vi "Script Example Project.vi"(8 "Error In":errorcluster, 10 "Hostname or IP":string="192.168.7.2", 11 "Device Name":string="BeagleBone Black") -> (0 "Error Out":errorcluster)   [LabVIEW 2019, in "LMH-LINX.lvlib"]
uses:
  <vilib>/MakerHub/LINX/LMH-LINX.lvlib
  <vilib>/MakerHub/Toolbox/LMH-Toolbox.lvlib
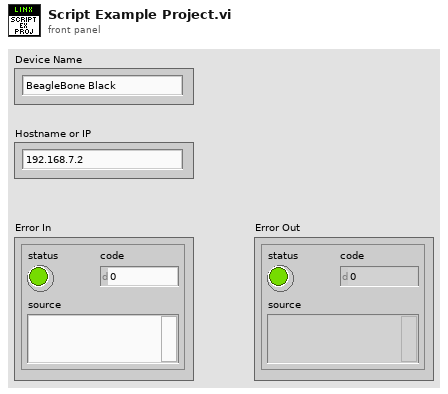
[diagram p1: front panel]
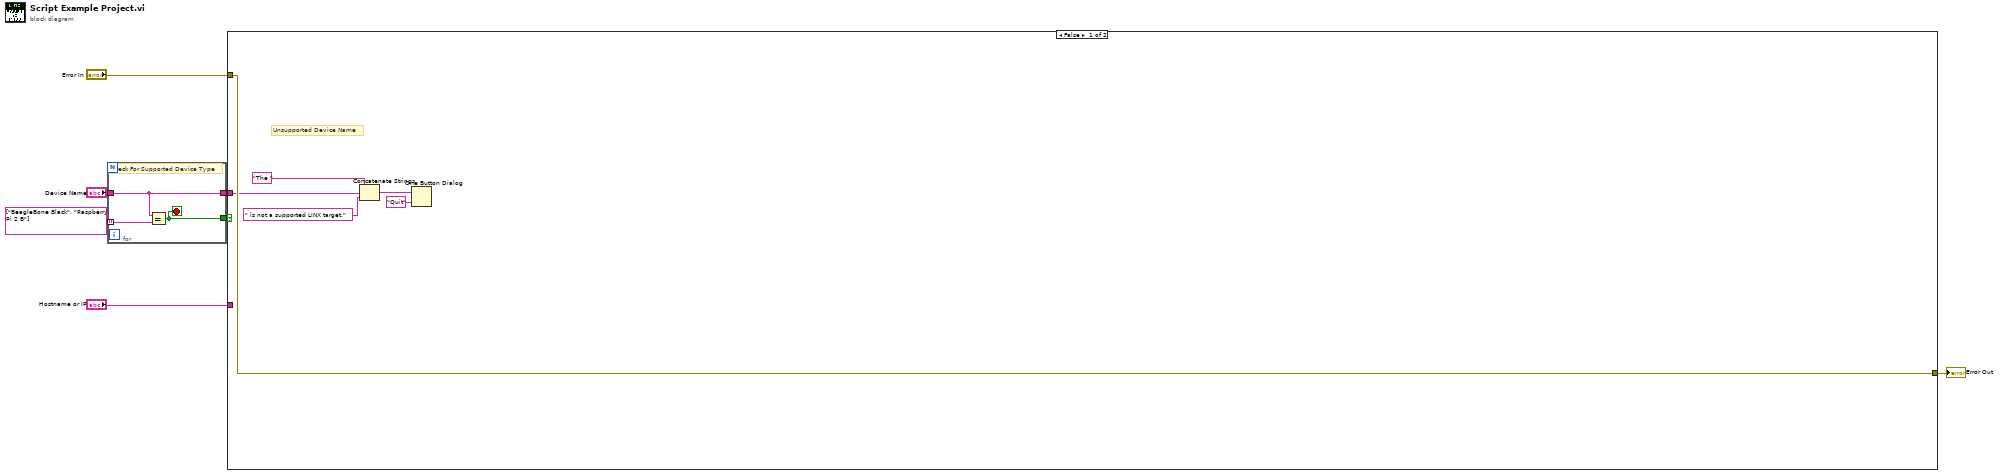
[diagram p0: block diagram]
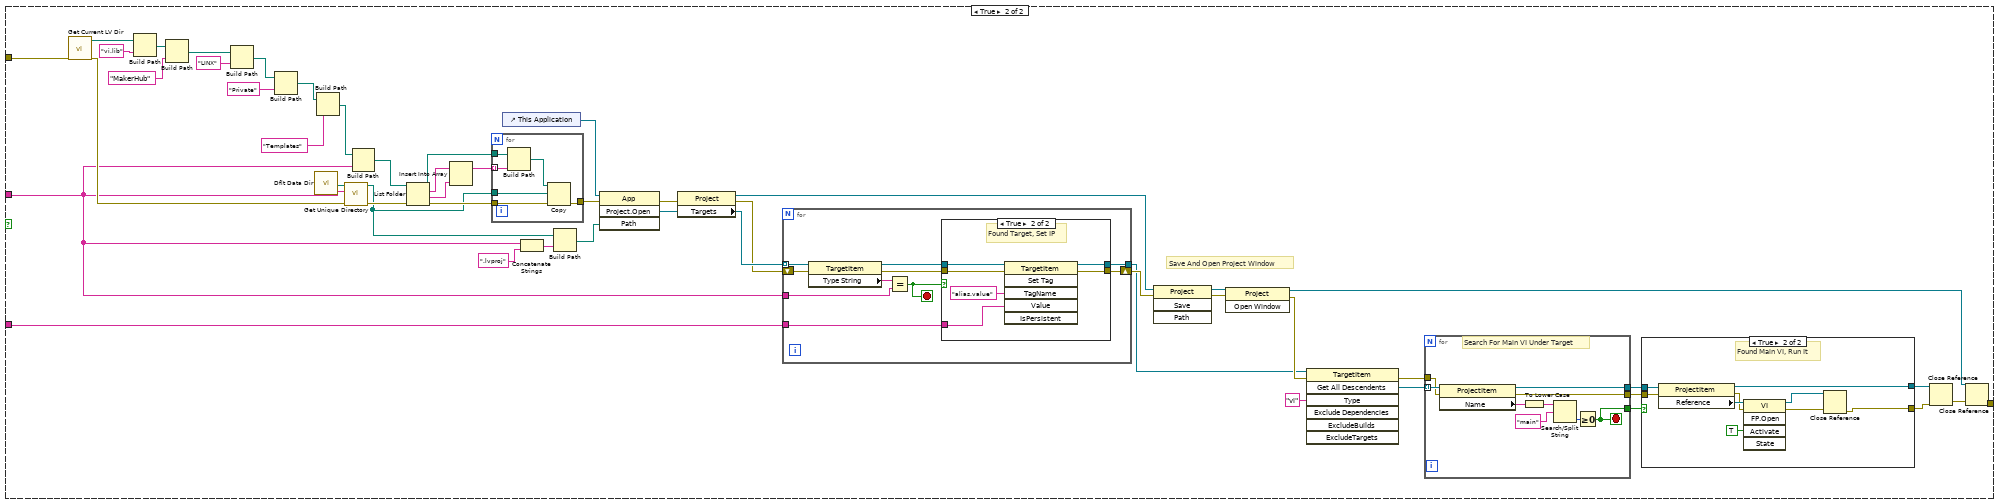
[diagram p2: hidden frame]
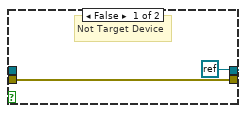
[diagram p4: hidden frame]
diagram:
  n1 = for {
    tunnel: string[] ["BeagleBone Black", "Raspberry Pi 2 B"] -> [w10] mode=indexing
    tunnel: "Device Name" -> [w8]
    tunnel: [w9] -> w1
    tunnel: [w8] -> w2
    stop <- w9 stop-if-true
    # "Check For Supported Device Type"
    n2 = Equal?(x=w8, y=w10) -> (x = y?=w9:bool)
  }
  n3 = case shown="False" w1 {
    tunnel: "Hostname or IP" -> [_ w53]
    tunnel: "Error In" -> [w16 w19]
    tunnel: [w16 w18] -> w5
    tunnel: w2 -> [w14 w17]
    frame False {
      # "Unsupported Device Name"
      n4 = Concatenate Strings("The " ("message"), w14, " is not a supported LINX target." ("string")) -> (w12:string)
      n5 = One Button Dialog(message=w12, button name ("OK")="Quit") -> ()  [unwired: 1 out]
    }
    frame True {
      # "Save And Open Project Window"
      n6 = call <vilib>:"Get Current LV Dir.vi"("Error In"=w19) -> ("Error Out"=w21:errorcluster, "This LV Directory"=w66:path)  [unwired: 9 in]
      n7 = Build Path(base path=w66, name or relative path="vi.lib") -> (appended path=w60:path)
      n8 = Build Path(base path=w60, name or relative path="MakerHub") -> (appended path=w59:path)
      n9 = Build Path(base path=w59, name or relative path="LINX") -> (appended path=w58:path)
      n10 = Build Path(base path=w58, name or relative path="Private") -> (appended path=w57:path)
      n11 = call <vilib>:"Dflt Data Dir.vi"() -> ("App:Default Data Directory"=w43:path)
      n12 = Build Path(base path=w57, name or relative path="Templates") -> (appended path=w56:path)
      n13 = call <vilib>:"Get Unique Directory.vi"("Error In"=w21, "Root Folder Name"=w17, "Parent Directory"=w43) -> ("Error Out"=w40:errorcluster, "Target Directory"=w35:path)  [unwired: 7 in]
      n14 = Build Path(base path=w56, name or relative path=w17) -> (appended path=w42:path)
      n15 = List Folder(path=w42, error in=w40) -> (path out=w37:path, filenames=w20:string[], folder names=w39:string[], error out=w41:errorcluster)  [unwired: 2 in]
      n16 = Insert Into Array(array=w20, new element=w39) -> (w38:string[])  [unwired: 1 in]
      n17 = for {
        tunnel: w41 -> [w92]
        tunnel: w38 -> [w91] mode=indexing
        tunnel: w37 -> [w90]
        tunnel: w35 -> [w88]
        tunnel: [w87] -> w36
        n18 = Build Path(base path=w90, name or relative path=w91) -> (appended path=w89:path)
        n19 = Copy(8:w92, 10:w88, 11:w89) -> (0:w87:errorcluster)  [unwired: 2 in, 2 out]
      }
      n20 = control-ref of="This Application"() -> (w22:refnum<vi>)
      n21 = Concatenate Strings(w17, ".lvproj" ("string")) -> (w45:string)
      n22 = Build Path(base path=w35, name or relative path=w45) -> (appended path=w46:path)
      n23 = invoke class="App" method="Project.Open"(reference=w22, error in=w36, "Path"=w46) -> (error out=w51:errorcluster, "Project:Open"=w55:refnum<vi>)  [unwired: 1 in, 2 out]
      n24 = property class="Project"(reference=w55, error in=w51) -> (reference out=w50:refnum<vi>, error out=w52:errorcluster, "Targets"=w54:refnum<vi>[])
      n25 = for {
        tunnel: w54 -> [w102] mode=indexing
        tunnel: w17 -> [w100]
        tunnel: w53 -> [w99]
        shift-right: [w94] -> w49
        shift-left: w52 -> [w95]
        tunnel: [w93] -> w33
        stop <- w98 stop-if-true
        n26 = property class="TargetItem"(reference=w102, error in=w95) -> (reference out=w97:refnum<vi>, error out=w96:errorcluster, "Type String"=w101:string)
        n27 = Equal?(x=w101, y=w100) -> (x = y?=w98:bool)
        n28 = case shown="True" w98 {
          tunnel: w99 -> [_ w109]
          tunnel: w97 -> [_ w108]
          tunnel: w96 -> [w104 w107]
          tunnel: [w104 w106] -> w94
          tunnel: [refnum<k0> refnum w105] -> w93
          frame False {
            # "Not Target Device"
          }
          frame True {
            # "Found Target, Set IP"
            n29 = invoke class="TargetItem" method="Set Tag"(reference=w108, error in=w107, "TagName"="alias.value", "Value"=w109) -> (reference out=w105:refnum<vi>, error out=w106:errorcluster)  [unwired: 2 in, 4 out]
          }
        }
      }
      n30 = invoke class="Project" method="Save"(reference=w50, error in=w49) -> (reference out=w48:refnum<vi>, error out=w47:errorcluster)  [unwired: 2 in, 2 out]
      n31 = invoke class="Project" method="Open Window"(reference=w48, error in=w47) -> (reference out=w23:refnum<vi>, error out=w34:errorcluster)  [unwired: 1 in, 1 out]
      n32 = invoke class="TargetItem" method="Get All Descendents"(reference=w33, error in=w34, "Type"="vi") -> (error out=w30:errorcluster, "All Descendents"=w31:refnum<vi>[])  [unwired: 4 in, 5 out]
      n33 = for {
        tunnel: w31 -> [w86] mode=indexing
        tunnel: w30 -> [w85]
        tunnel: [w80] -> w29
        tunnel: [w79] -> w28
        tunnel: [w78] -> w27
        stop <- w80 stop-if-true
        # "Search For Main VI Under Target"
        n34 = property class="ProjectItem"(reference=w86, error in=w85) -> (reference out=w79:refnum<vi>, error out=w78:errorcluster, "Name"=w84:string)
        n35 = To Lower Case(string=w84) -> (all lower case string=w83:string)
        n36 = Search/Split String(string=w83, search string/char (-)="main") -> (offset of match=w81:i32)  [unwired: 1 in, 2 out]
        n37 = Greater Or Equal To 0?(x=w81) -> (x >= 0?=w80:bool)
      }
      n38 = case shown="True" w29 {
        tunnel: w28 -> [w67 w77]
        tunnel: w27 -> [w68 w76]
        tunnel: [w68 w69] -> w26
        tunnel: [w67 w72] -> w25
        frame False {
        }
        frame True {
          # "Found Main VI, Run It"
          n39 = property class="ProjectItem"(reference=w77, error in=w76) -> (reference out=w72:refnum<vi>, error out=w74:errorcluster, "Reference"=w75:refnum<vi>)
          n40 = invoke class="VI" method="FP.Open"(reference=w75, error in=w74, "Activate"=TRUE ("Activate?")) -> (reference out=w70:refnum<vi>, error out=w71:errorcluster)  [unwired: 2 in, 3 out]
          n41 = Close Reference(reference=w70, error in (no error)=w71) -> (error out=w69:errorcluster)
        }
      }
      n42 = Close Reference(reference=w25, error in (no error)=w26) -> (error out=w24:errorcluster)
      n43 = Close Reference(reference=w23, error in (no error)=w24) -> (error out=w18:errorcluster)
    }
  }
  "Error Out" <- w5
